vi "1.Basic demo.vi"() -> ()   [LabVIEW 2020]
uses:
  UnderAutomation.UniversalRobots/UnderAutomation.UniversalRobots.lvlib
  C:/Users/fg/Documents/UniversalRobots.vi/LabVIEW_2024/UnderAutomation.UniversalRobots/lib/UnderAutomation.UniversalRobots.dll
  LabVIEW_2024/UnderAutomation.UniversalRobots/lib/UnderAutomation.UniversalRobots.dll
panel:
  out "Response":cluster{"Message":string, "Succeed":bool}
  in  "OK Button":bool
  out "Configurable0":bool
  out "error out":errorcluster
  out "Waveform 1":dbl(graph)
  out "Connected":bool
  in  "stop":bool
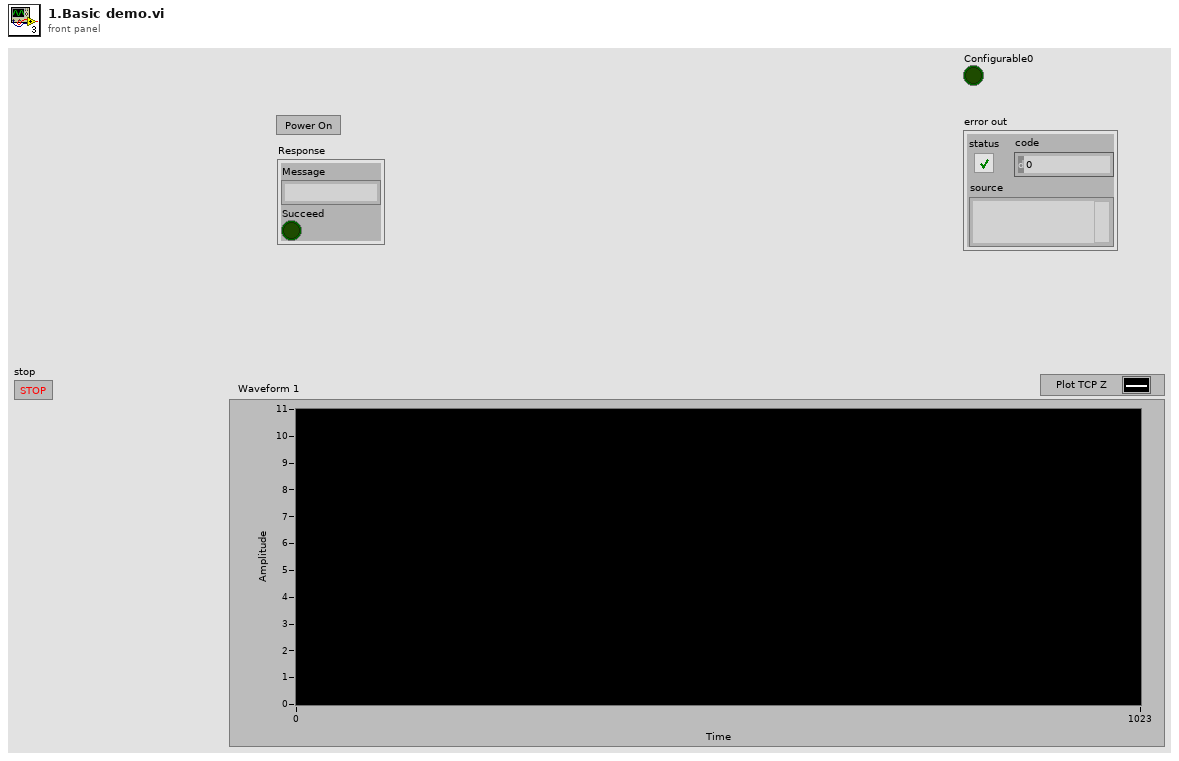
[diagram p1: front panel]
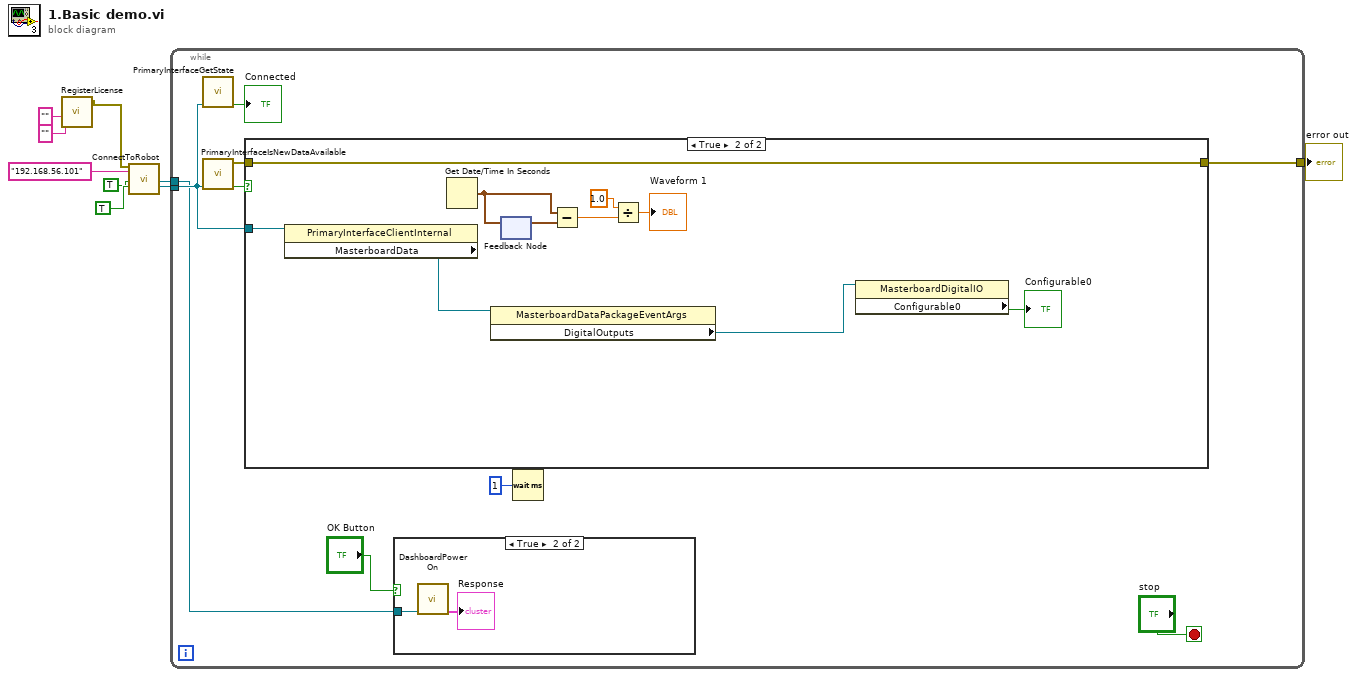
[diagram p0: block diagram]
diagram:
  n1 = call "RegisterLicense.vi"("key"="", "licensee"="") -> ("error out"=w5:errorcluster)  [unwired: 6 in, 2 out]
  n2 = call "ConnectToRobot.vi"("error in"=w5, "ip"="192.168.56.101", "Enable Dashboard"=TRUE ("Enable Primary Interface"), "Enable Primary Interface"=TRUE) -> ("Dashboard"=w2:refnum<k24>, "PrimaryInterface"=w6:refnum<k24>)  [unwired: 10 in, 4 out]
  n3 = while {
    tunnel: w6 -> [w14]
    tunnel: [w12] -> w7
    tunnel: w2 -> [w11]
    stop <- "stop" stop-if-true
    n4 = call "PrimaryInterfaceGetState.vi"("PrimaryInterface"=w14) -> ("Connected"=→"Connected":bool)  [unwired: 9 in, 1 out]
    n5 = call "PrimaryInterfaceIsNewDataAvailable.vi"("PrimaryInterface"=w14) -> ("Data available"=w15:bool, "error out"=w13:errorcluster)  [unwired: 9 in]
    n6 = case shown="True" w15 {
      tunnel: w14 -> [_ w26]
      tunnel: w13 -> [w21 w24]
      tunnel: [w21 w24] -> w12
      frame False {
      }
      frame True {
        n7 = property class="PrimaryInterfaceClientInternal"(reference=w26) -> ("MasterboardData"=w25:refnum<k24>)  [unwired: 1 in, 2 out]
        n8 = Get Date/Time In Seconds() -> (seconds since 1Jan1904=w31:timestamp)
        n9 = property class="MasterboardDataPackageEventArgs"(reference=w25) -> ("DigitalOutputs"=w22:refnum<k24>)  [unwired: 1 in, 2 out]
        n10 = feedback #1() -> (w30:timestamp)  [unwired: 1 in]
        n11 = feedback-in #1(w31) -> ()
        n12 = Subtract(x=w31, y=w30) -> (x-y=w29:dbl)
        n13 = Divide(x=1.0, y=w29) -> (x/y=→"Waveform 1":dbl)
        n14 = property class="MasterboardDigitalIO"(reference=w22) -> ("Configurable0"=→"Configurable0":bool)  [unwired: 1 in, 2 out]
      }
    }
    n15 = case shown="True" "OK Button" {
      tunnel: w11 -> [_ w20]
      frame False {
      }
      frame True {
        n16 = call "DashboardPowerOn.vi"("Dashboard"=w20) -> ("Response"=→"Response":cluster{"Message":string, "Succeed":bool})  [unwired: 9 in, 1 out]
      }
    }
    n17 = Wait (ms)(milliseconds to wait=u32 1) -> ()  [unwired: 1 out]
  }
  "error out" <- w7
